vi "image.vi"() -> ()   [LabVIEW 2012]
uses:
  <vilib>/picture/picture.llb/imagedata.ctl
  <vilib>/Analysis/2dsp.llb/2D Convolution (DBL).vi
  <vilib>/picture/picture.llb/Draw True-Color Pixmap.vi
  <vilib>/Analysis/NI_AALPro.lvlib
panel:
  out "new picture 3":picture
  out "new picture 2":picture
  out "new picture":picture
  out "image data":T1
  in  "Path":path
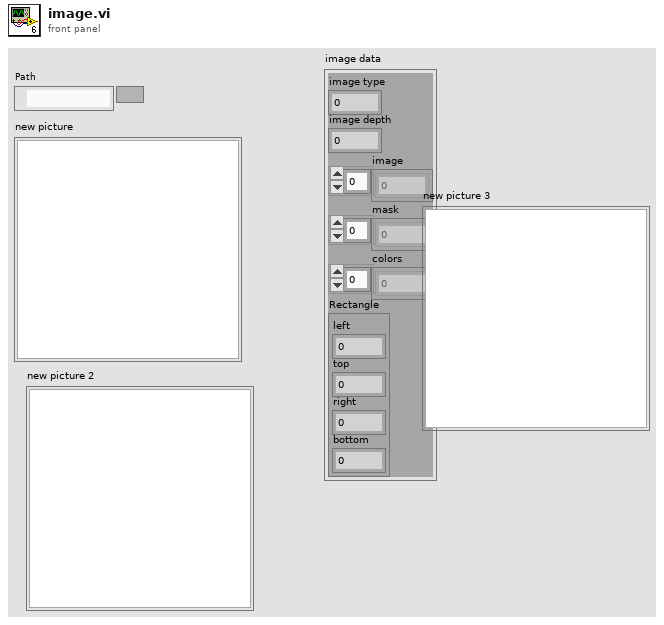
[diagram p1: front panel]
types:
  T1 = typedef "imagedata.ctl" = cluster{"image type":i32, "image depth":i32, "image":u8[], "mask":u8[], "colors":u32[], "Rectangle":cluster{"left":i16, "top":i16, "right":i16, "bottom":i16}}
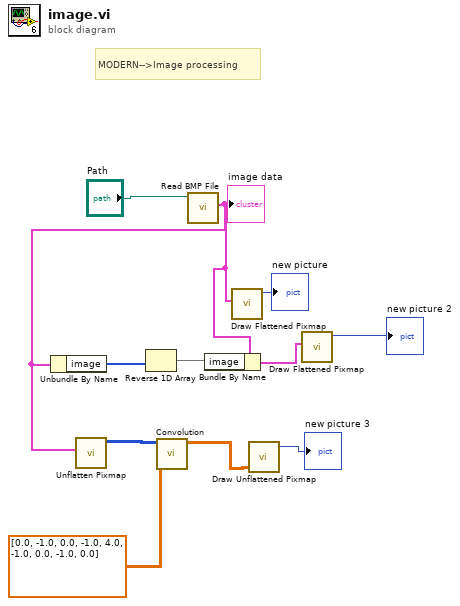
[diagram p0: block diagram]
diagram:
  # "MODERN-->Image processing"
  n1 = call <vilib>:"Read BMP File.vi"("path to BMP file"="Path") -> ("image data"=w5:T1)  [unwired: 8 in, 2 out]
  "image data" <- w5
  n2 = Unbundle By Name(w5) -> ("image"=w9:u8[])
  n3 = call <vilib>:"Unflatten Pixmap.vi"("image data"=w5) -> ("24-bit pixmap"=w4:u32[][])  [unwired: 4 in, 6 out]
  n4 = Reverse 1D Array(array=w9) -> (reversed array=w8:u8[])
  n5 = call-poly <vilib>:"Convolution.vi"("Y"=dbl[][] [[0.0, -1.0, 0.0], [-1.0, 4.0, -1.0], [0.0, -1.0, 0.0]], "X"=w4) -> ("X * Y"=w2:dbl[][])  [unwired: 8 in, 1 out]
  n6 = Bundle By Name(cluster=w5, "image"=w8) -> (w7:T1)
  n7 = call <vilib>:"Draw Flattened Pixmap.vi"("image data"=w5) -> ("new picture"=→"new picture":picture)  [unwired: 8 in]
  n8 = call-poly <vilib>:"Draw Unflattened Pixmap.vi"("data (RGB format)"=w2) -> ("new picture"=→"new picture 3":picture)  [unwired: 8 in]
  n9 = call <vilib>:"Draw Flattened Pixmap.vi"("image data"=w7) -> ("new picture"=→"new picture 2":picture)  [unwired: 8 in]
